vi "Set_PScontrol_backup.vi"(7 "Magnet PS":u16(ring) items=["Resistive Magnet", "SCM2", "SCM1", "Generic SC power supply", "PPMS"], 8 "error in (no error)":errorcluster, 9 "PS Control VI Name":string="PS Control.vi", 10 "Command_Message_in":T2, 11 "Command_queue_in":T1) -> (0 "error out":errorcluster, 2 "Command_Message_out":T2, 3 "Command_queue_out":T1)   [LabVIEW 2025]
uses:
  Command_Message.ctl
  Command_Queue.ctl
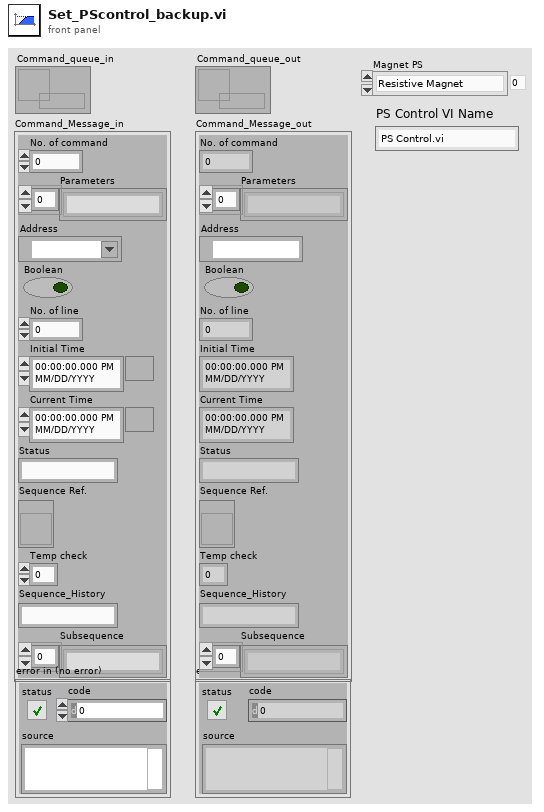
[diagram p1: front panel]
types:
  T1 = typedef "Command_Queue.ctl" = refnum<queue>
  T2 = typedef "Command_Message.ctl" = cluster{"No. of command":i32, "Parameters":string[], "Address":refnum<visa-resource-name>, "Boolean":bool, "No. of line":i32, "Initial Time":timestamp, "Current Time":timestamp, "Status":string, "Sequence Ref.":refnum<vi>, "Temp check":i32, "Sequence_History":string, "Subsequence":string[]}
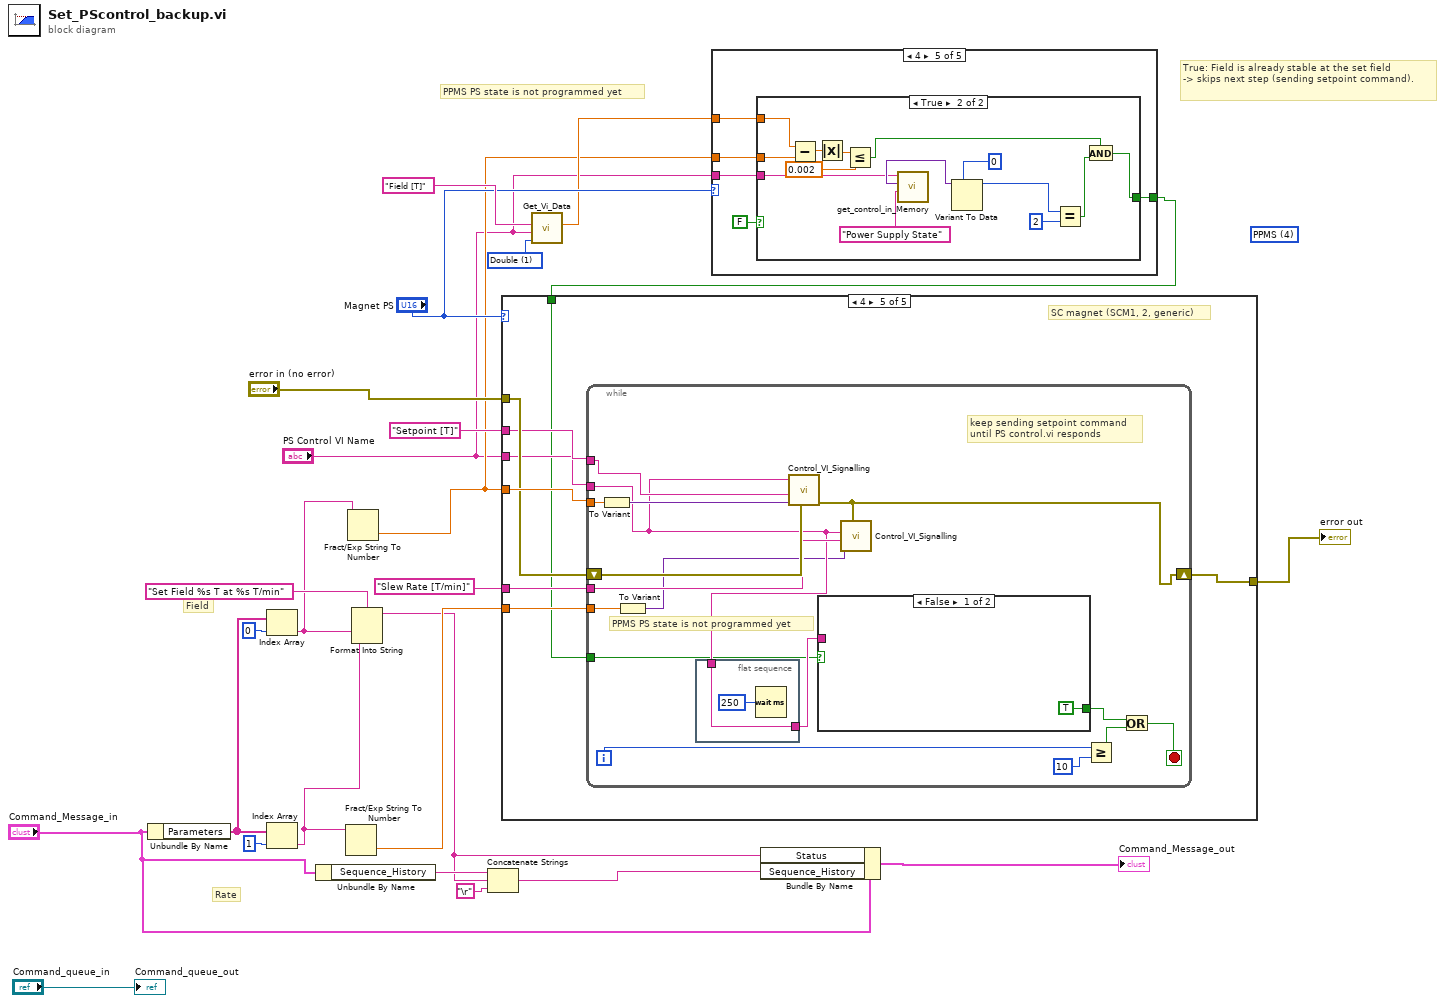
[diagram p0: block diagram]
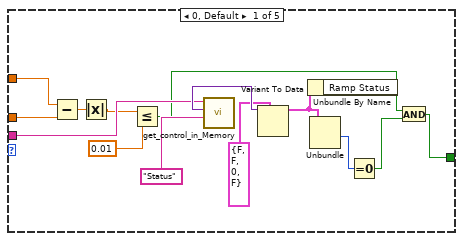
[diagram p2: hidden frame]
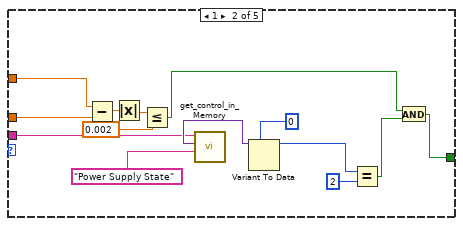
[diagram p3: hidden frame]
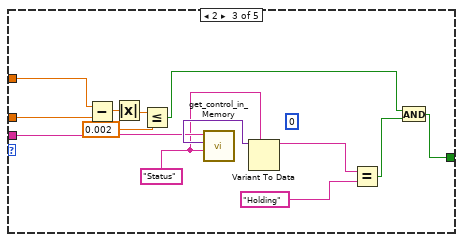
[diagram p4: hidden frame]
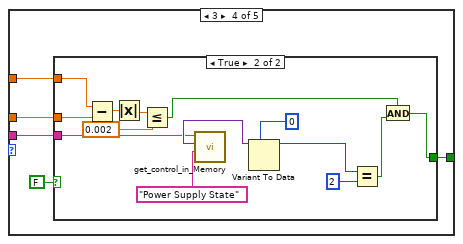
[diagram p5: hidden frame]
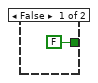
[diagram p6: hidden frame]
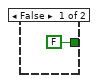
[diagram p7: hidden frame]
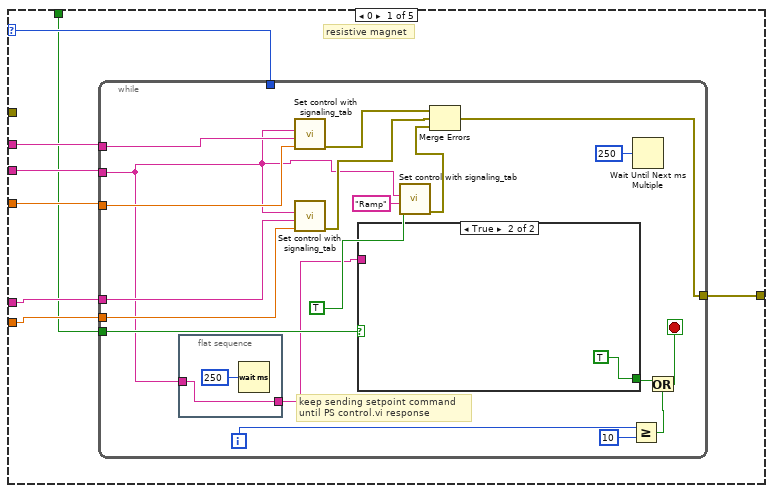
[diagram p8: hidden frame]
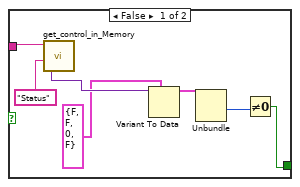
[diagram p9: hidden frame]
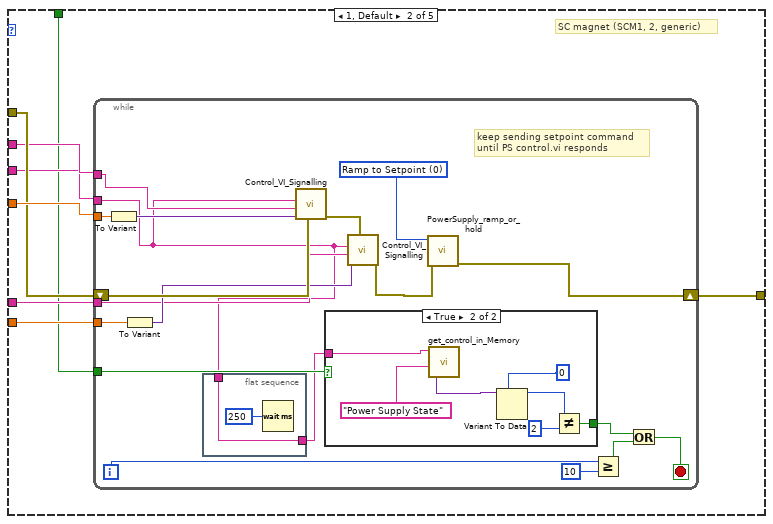
[diagram p10: hidden frame]
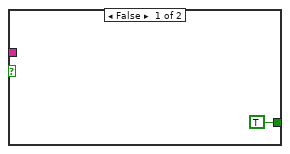
[diagram p11: hidden frame]
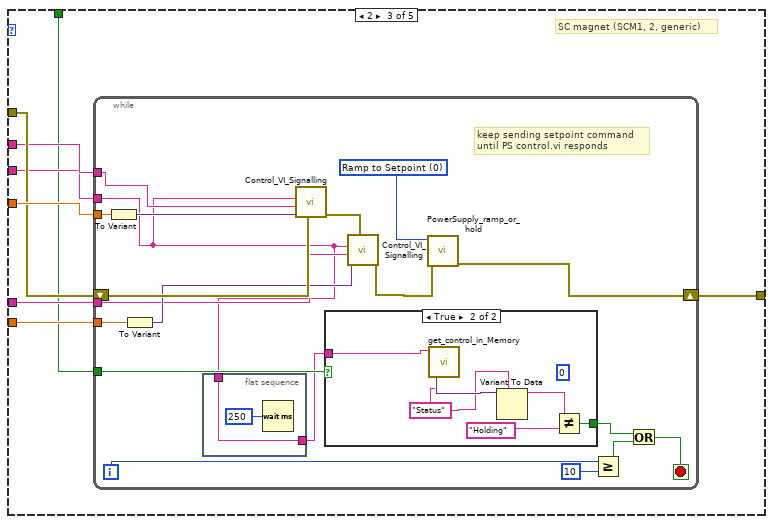
[diagram p12: hidden frame]
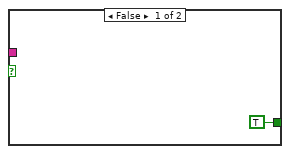
[diagram p13: hidden frame]
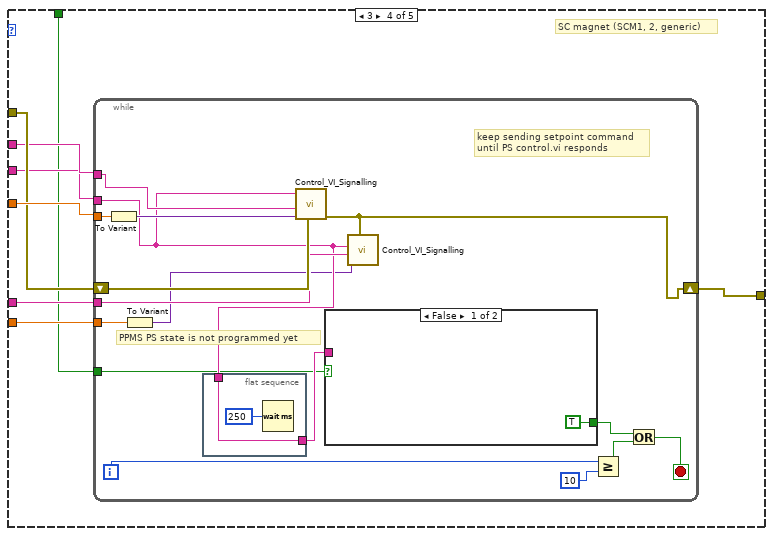
[diagram p14: hidden frame]
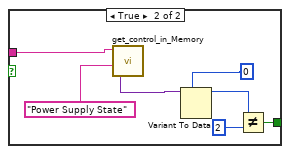
[diagram p15: hidden frame]
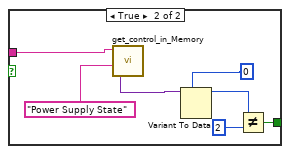
[diagram p16: hidden frame]
diagram:
  (unwired) u16 4 items=["Resistive Magnet", "SCM2", "SCM1", "Generic SC power supply", "PPMS"] ("Magnet PS")
  w5 = u16 1 items=["String", "Double", "Boolean", "Variant"] ("Data Type")
  # "PPMS PS state is not programmed yet"
  # "True: Field is already stable at the set field\n-> skips next step (sending setpoint command)."
  # "Rate"
  # "Field"
  n1 = Unbundle By Name("Command_Message_in") -> ("Parameters"=w16:string[])
  n2 = Index Array(array=w16, index=0) -> (element=w19:string)
  n3 = Index Array(array=w16, index=1) -> (element=w18:string)
  n4 = Unbundle By Name("Command_Message_in") -> ("Sequence_History"=w13:string)
  n5 = Fract/Exp String To Number(string=w18) -> (number=w22:dbl)  [unwired: 3 in, 1 out]
  n6 = Fract/Exp String To Number(string=w19) -> (number=w3:dbl)  [unwired: 3 in, 1 out]
  n7 = Format Into String(format string="Set Field %s T at %s T/min", w19, w18) -> (resulting string=w12:string)  [unwired: 2 in, 1 out]
  n8 = Concatenate Strings(w13, w12, "\r") -> (w10:string)
  n9 = call "Get_Vi_Data.vi"("Data Type"=w5, "VI name"="PS Control VI Name", "Control Name"="Field [T]") -> ("Data (Double)"=w4:dbl)  [unwired: 4 in, 4 out]
  n10 = case shown="4" "Magnet PS" {
    tunnel: "PS Control VI Name" -> [w37 w50 w65 w71 w91]
    tunnel: [w36 w46 w62 w70 w90] -> w2
    tunnel: w4 -> [w35 w45 w61 w69 w89]
    tunnel: w3 -> [w34 w44 w60 w68 w88]
    frame 0, Default {
      n11 = Subtract(x=w35, y=w34) -> (x-y=w33:dbl)
      n12 = Absolute Value(x=w33) -> (abs(x)=w29:dbl)
      n13 = Less Or Equal?(x=w29, y=0.01) -> (x <= y?=w31:bool)
      n14 = call "get_control_in_Memory.vi"("Control Name"="Status", "VI Name"=w37) -> ("Value"=w38:variant)  [unwired: 2 in, 1 out]
      n15 = Variant To Data(type=cluster{bool, bool, "Ramp Status":u16, bool} {FALSE, FALSE, "Ramp Status"=0, FALSE} ("Status"), Variant=w38) -> (data=w28:cluster{bool, bool, "Ramp Status":u16, bool})  [unwired: 1 in, 1 out]
      n16 = Unbundle By Name(w28) -> ()  [unwired: 1 out]
      n17 = Unbundle(w28) -> ("Ramp Status"=w27:u16)  [unwired: 3 out]
      n18 = Equal To 0?(x=w27) -> (x = 0?=w26:bool)
      n19 = And(x=w31, y=w26) -> (x .and. y?=w36:bool)
    }
    frame 1 {
      n20 = Subtract(x=w45, y=w44) -> (x-y=w43:dbl)
      n21 = Absolute Value(x=w43) -> (abs(x)=w40:dbl)
      n22 = Less Or Equal?(x=w40, y=0.002) -> (x <= y?=w41:bool)
      n23 = call "get_control_in_Memory.vi"("Control Name"="Power Supply State", "VI Name"=w50) -> ("Value"=w52:variant)  [unwired: 2 in, 1 out]
      n24 = Variant To Data(type=0, Variant=w52) -> (data=w48:i32)  [unwired: 1 in, 1 out]
      n25 = Equal?(x=w48, y=2) -> (x = y?=w47:bool)
      n26 = And(x=w41, y=w47) -> (x .and. y?=w46:bool)
    }
    frame 2 {
      (unwired) 0
      w55 = "Status" ("Control Name")
      n27 = Subtract(x=w61, y=w60) -> (x-y=w59:dbl)
      n28 = Absolute Value(x=w59) -> (abs(x)=w56:dbl)
      n29 = Less Or Equal?(x=w56, y=0.002) -> (x <= y?=w57:bool)
      n30 = call "get_control_in_Memory.vi"("Control Name"=w55, "VI Name"=w65) -> ("Value"=w66:variant)  [unwired: 2 in, 1 out]
      n31 = Variant To Data(type=w55, Variant=w66) -> (data=w64:string)  [unwired: 1 in, 1 out]
      n32 = Equal?(x=w64, y="Holding" ("Control Name")) -> (x = y?=w63:bool)
      n33 = And(x=w57, y=w63) -> (x .and. y?=w62:bool)
    }
    frame 3 {
      n34 = case shown="True" FALSE {
        tunnel: w71 -> [_ w83]
        tunnel: [FALSE w79] -> w70
        tunnel: w69 -> [_ w78]
        tunnel: w68 -> [_ w77]
        frame False {
        }
        frame True {
          n35 = Subtract(x=w78, y=w77) -> (x-y=w76:dbl)
          n36 = Absolute Value(x=w76) -> (abs(x)=w73:dbl)
          n37 = Less Or Equal?(x=w73, y=0.002) -> (x <= y?=w74:bool)
          n38 = call "get_control_in_Memory.vi"("Control Name"="Power Supply State", "VI Name"=w83) -> ("Value"=w85:variant)  [unwired: 2 in, 1 out]
          n39 = Variant To Data(type=0, Variant=w85) -> (data=w81:i32)  [unwired: 1 in, 1 out]
          n40 = Equal?(x=w81, y=2) -> (x = y?=w80:bool)
          n41 = And(x=w74, y=w80) -> (x .and. y?=w79:bool)
        }
      }
    }
    frame 4 {
      n42 = case shown="True" FALSE {
        tunnel: w91 -> [_ w103]
        tunnel: [FALSE w99] -> w90
        tunnel: w89 -> [_ w98]
        tunnel: w88 -> [_ w97]
        frame False {
        }
        frame True {
          n43 = Subtract(x=w98, y=w97) -> (x-y=w96:dbl)
          n44 = Absolute Value(x=w96) -> (abs(x)=w93:dbl)
          n45 = Less Or Equal?(x=w93, y=0.002) -> (x <= y?=w94:bool)
          n46 = call "get_control_in_Memory.vi"("Control Name"="Power Supply State", "VI Name"=w103) -> ("Value"=w105:variant)  [unwired: 2 in, 1 out]
          n47 = Variant To Data(type=0, Variant=w105) -> (data=w101:i32)  [unwired: 1 in, 1 out]
          n48 = Equal?(x=w101, y=2) -> (x = y?=w100:bool)
          n49 = And(x=w94, y=w100) -> (x .and. y?=w99:bool)
        }
      }
    }
  }
  n50 = case shown="4" "Magnet PS" {
    selector: "Magnet PS" -> [w108 _ _ _ _]
    tunnel: w3 -> [w110 w151 w188 w224 w258]
    tunnel: "error in (no error)" -> [_ w150 w187 w223 w257]
    tunnel: w22 -> [w109 w149 w186 w222 w256]
    tunnel: [w114 w148 w185 w221 w255] -> w21
    tunnel: "Setpoint [T]" -> [w113 w147 w184 w220 w254]
    tunnel: "PS Control VI Name" -> [w112 w145 w182 w218 w252]
    tunnel: "Slew Rate [T/min]" ("Control Name") -> [w111 w146 w183 w219 w253]
    tunnel: w2 -> [w107 w144 w181 w217 w251]
    frame 0 {
      # "resistive magnet"
      n51 = while {
        tunnel: [w118] -> w114
        tunnel: w113 -> [w128]
        tunnel: w112 -> [w116]
        tunnel: w111 -> [w127]
        tunnel: w110 -> [w126]
        tunnel: w109 -> [w125]
        tunnel: w108 -> [_]
        tunnel: w107 -> [w117]
        i -> [w123]
        stop <- w119 stop-if-true
        # "keep sending setpoint command\nuntil PS control.vi response"
        n52 = flat-sequence {
          tunnel: [w134] -> w115
          tunnel: w116 -> [w134]
          frame #0 {
            n53 = Wait (ms)(milliseconds to wait=u32 250) -> ()  [unwired: 1 out]
          }
        }
        n54 = call "Set control with signaling_tab.vi"("Value (Signaling)"=w126, "Control Name"=w128, "VI Name"=w116) -> ("error out"=w131:errorcluster)  [unwired: 8 in]
        n55 = call "Set control with signaling_tab.vi"("Value (Signaling)"=w125, "Control Name"=w127, "VI Name"=w116) -> ("error out"=w130:errorcluster)  [unwired: 8 in]
        n56 = case shown="True" w117 {
          tunnel: w115 -> [w137 _]
          tunnel: [w136 TRUE] -> w121
          frame False {
            n57 = call "get_control_in_Memory.vi"("Control Name"="Status", "VI Name"=w137) -> ("Value"=w141:variant)  [unwired: 2 in, 1 out]
            n58 = Variant To Data(type=cluster{bool, bool, "Ramp Status":u16, bool} {FALSE, FALSE, "Ramp Status"=0, FALSE} ("Status"), Variant=w141) -> (data=w142:cluster{bool, bool, "Ramp Status":u16, bool})  [unwired: 1 in, 1 out]
            n59 = Unbundle(w142) -> ("Ramp Status"=w138:u16)  [unwired: 3 out]
            n60 = Not Equal To 0?(x=w138) -> (x != 0?=w136:bool)
          }
          frame True {
          }
        }
        n61 = call "Set control with signaling_tab.vi"("Value (Signaling)"=TRUE, "Control Name"="Ramp", "VI Name"=w116) -> ("error out"=w129:errorcluster)  [unwired: 8 in]
        n62 = Merge Errors(w131, w130, w129) -> (w118:errorcluster)
        n63 = Greater Or Equal?(x=w123, y=10) -> (x >= y?=w120:bool)
        n64 = Wait Until Next ms Multiple(millisecond multiple=u32 250) -> ()  [unwired: 1 out]
        n65 = Or(x=w121, y=w120) -> (x .or. y?=w119:bool)
      }
    }
    frame 1, Default {
      # "SC magnet (SCM1, 2, generic)"
      n66 = while {
        tunnel: w151 -> [w170]
        tunnel: w149 -> [w166]
        tunnel: w147 -> [w161]
        tunnel: w145 -> [w152]
        tunnel: w146 -> [w160]
        shift-right: [w162] -> w148
        shift-left: w150 -> [w168]
        tunnel: w144 -> [w154]
        i -> [w159]
        stop <- w155 stop-if-true
        w163 = u16 0 items=["Ramp to Setpoint", "Hold"] ("Mode")
        # "keep sending setpoint command\nuntil PS control.vi responds"
        n67 = To Variant(anything=w170) -> (Variant=w169:variant)
        n68 = To Variant(anything=w166) -> (Variant=w165:variant)
        n69 = flat-sequence {
          tunnel: [w171] -> w153
          tunnel: w152 -> [w171]
          frame #0 {
            n70 = Wait (ms)(milliseconds to wait=u32 250) -> ()  [unwired: 1 out]
          }
        }
        n71 = call "Control_VI_Signalling.vi"("error in (no error)"=w168, "Input Value"=w169, "Control Name"=w161, "Target VI name"=w152) -> ("error out"=w167:errorcluster)  [unwired: 7 in]
        n72 = case shown="True" w154 {
          tunnel: [TRUE w175] -> w157
          tunnel: w153 -> [_ w174]
          frame False {
          }
          frame True {
            n73 = call "get_control_in_Memory.vi"("Control Name"="Power Supply State", "VI Name"=w174) -> ("Value"=w179:variant)  [unwired: 2 in, 1 out]
            n74 = Variant To Data(type=0, Variant=w179) -> (data=w177:i32)  [unwired: 1 in, 1 out]
            n75 = Not Equal?(x=w177, y=2) -> (x != y?=w175:bool)
          }
        }
        n76 = call "Control_VI_Signalling.vi"("error in (no error)"=w167, "Input Value"=w165, "Control Name"=w160, "Target VI name"=w152) -> ("error out"=w164:errorcluster)  [unwired: 7 in]
        n77 = call "PowerSupply_ramp_or_hold.vi"("error in (no error)"=w164, "Mode"=w163) -> ("error out"=w162:errorcluster)  [unwired: 9 in]
        n78 = Greater Or Equal?(x=w159, y=10) -> (x >= y?=w156:bool)
        n79 = Or(x=w157, y=w156) -> (x .or. y?=w155:bool)
      }
    }
    frame 2 {
      # "SC magnet (SCM1, 2, generic)"
      n80 = while {
        tunnel: w188 -> [w207]
        tunnel: w186 -> [w203]
        tunnel: w184 -> [w198]
        tunnel: w182 -> [w189]
        tunnel: w183 -> [w197]
        shift-right: [w199] -> w185
        shift-left: w187 -> [w205]
        tunnel: w181 -> [w191]
        i -> [w196]
        stop <- w192 stop-if-true
        w200 = u16 0 items=["Ramp to Setpoint", "Hold"] ("Mode")
        # "keep sending setpoint command\nuntil PS control.vi responds"
        n81 = To Variant(anything=w207) -> (Variant=w206:variant)
        n82 = To Variant(anything=w203) -> (Variant=w202:variant)
        n83 = flat-sequence {
          tunnel: [w208] -> w190
          tunnel: w189 -> [w208]
          frame #0 {
            n84 = Wait (ms)(milliseconds to wait=u32 250) -> ()  [unwired: 1 out]
          }
        }
        n85 = call "Control_VI_Signalling.vi"("error in (no error)"=w205, "Input Value"=w206, "Control Name"=w198, "Target VI name"=w189) -> ("error out"=w204:errorcluster)  [unwired: 7 in]
        n86 = case shown="True" w191 {
          tunnel: [TRUE w214] -> w194
          tunnel: w190 -> [_ w213]
          frame False {
          }
          frame True {
            (unwired) 0
            w212 = "Status" ("Control Name")
            n87 = call "get_control_in_Memory.vi"("Control Name"=w212, "VI Name"=w213) -> ("Value"=w216:variant)  [unwired: 2 in, 1 out]
            n88 = Variant To Data(type=w212, Variant=w216) -> (data=w215:string)  [unwired: 1 in, 1 out]
            n89 = Not Equal?(x=w215, y="Holding" ("Control Name")) -> (x != y?=w214:bool)
          }
        }
        n90 = call "Control_VI_Signalling.vi"("error in (no error)"=w204, "Input Value"=w202, "Control Name"=w197, "Target VI name"=w189) -> ("error out"=w201:errorcluster)  [unwired: 7 in]
        n91 = call "PowerSupply_ramp_or_hold.vi"("error in (no error)"=w201, "Mode"=w200) -> ("error out"=w199:errorcluster)  [unwired: 9 in]
        n92 = Greater Or Equal?(x=w196, y=10) -> (x >= y?=w193:bool)
        n93 = Or(x=w194, y=w193) -> (x .or. y?=w192:bool)
      }
    }
    frame 3 {
      # "SC magnet (SCM1, 2, generic)"
      n94 = while {
        tunnel: w224 -> [w240]
        tunnel: w222 -> [w237]
        tunnel: w220 -> [w236]
        tunnel: w218 -> [w233]
        tunnel: w219 -> [w235]
        shift-right: [w232] -> w221
        shift-left: w223 -> [w238]
        tunnel: w217 -> [w226]
        i -> [w234]
        stop <- w225 stop-if-true
        # "PPMS PS state is not programmed yet"
        # "keep sending setpoint command\nuntil PS control.vi responds"
        n95 = To Variant(anything=w240) -> (Variant=w239:variant)
        n96 = To Variant(anything=w237) -> (Variant=w231:variant)
        n97 = flat-sequence {
          tunnel: [w241] -> w227
          tunnel: w233 -> [w241]
          frame #0 {
            n98 = Wait (ms)(milliseconds to wait=u32 250) -> ()  [unwired: 1 out]
          }
        }
        n99 = call "Control_VI_Signalling.vi"("error in (no error)"=w238, "Input Value"=w239, "Control Name"=w236, "Target VI name"=w233) -> ("error out"=w232:errorcluster)  [unwired: 7 in]
        n100 = case shown="False" w226 {
          tunnel: [TRUE w245] -> w229
          tunnel: w227 -> [_ w244]
          frame False {
          }
          frame True {
            n101 = call "get_control_in_Memory.vi"("Control Name"="Power Supply State", "VI Name"=w244) -> ("Value"=w249:variant)  [unwired: 2 in, 1 out]
            n102 = Variant To Data(type=0, Variant=w249) -> (data=w247:i32)  [unwired: 1 in, 1 out]
            n103 = Not Equal?(x=w247, y=2) -> (x != y?=w245:bool)
          }
        }
        n104 = call "Control_VI_Signalling.vi"("error in (no error)"=w232, "Input Value"=w231, "Control Name"=w235, "Target VI name"=w233) -> ()  [unwired: 7 in, 1 out]
        n105 = Greater Or Equal?(x=w234, y=10) -> (x >= y?=w228:bool)
        n106 = Or(x=w229, y=w228) -> (x .or. y?=w225:bool)
      }
    }
    frame 4 {
      # "SC magnet (SCM1, 2, generic)"
      n107 = while {
        tunnel: w258 -> [w274]
        tunnel: w256 -> [w271]
        tunnel: w254 -> [w270]
        tunnel: w252 -> [w267]
        tunnel: w253 -> [w269]
        shift-right: [w266] -> w255
        shift-left: w257 -> [w272]
        tunnel: w251 -> [w260]
        i -> [w268]
        stop <- w259 stop-if-true
        # "PPMS PS state is not programmed yet"
        # "keep sending setpoint command\nuntil PS control.vi responds"
        n108 = To Variant(anything=w274) -> (Variant=w273:variant)
        n109 = To Variant(anything=w271) -> (Variant=w265:variant)
        n110 = flat-sequence {
          tunnel: [w275] -> w261
          tunnel: w267 -> [w275]
          frame #0 {
            n111 = Wait (ms)(milliseconds to wait=u32 250) -> ()  [unwired: 1 out]
          }
        }
        n112 = call "Control_VI_Signalling.vi"("error in (no error)"=w272, "Input Value"=w273, "Control Name"=w270, "Target VI name"=w267) -> ("error out"=w266:errorcluster)  [unwired: 7 in]
        n113 = case shown="False" w260 {
          tunnel: [TRUE w279] -> w263
          tunnel: w261 -> [_ w278]
          frame False {
          }
          frame True {
            n114 = call "get_control_in_Memory.vi"("Control Name"="Power Supply State", "VI Name"=w278) -> ("Value"=w283:variant)  [unwired: 2 in, 1 out]
            n115 = Variant To Data(type=0, Variant=w283) -> (data=w281:i32)  [unwired: 1 in, 1 out]
            n116 = Not Equal?(x=w281, y=2) -> (x != y?=w279:bool)
          }
        }
        n117 = call "Control_VI_Signalling.vi"("error in (no error)"=w266, "Input Value"=w265, "Control Name"=w269, "Target VI name"=w267) -> ()  [unwired: 7 in, 1 out]
        n118 = Greater Or Equal?(x=w268, y=10) -> (x >= y?=w262:bool)
        n119 = Or(x=w263, y=w262) -> (x .or. y?=w259:bool)
      }
    }
  }
  "error out" <- w21
  n120 = Bundle By Name(cluster="Command_Message_in", "Status"=w12, "Sequence_History"=w10) -> (→"Command_Message_out":T2)
  "Command_queue_out" <- "Command_queue_in"
